vi "proc_get_exit_code.vi"(8 "error in":errorcluster, 10 "ignore error":bool=TRUE, 11 "process instance handle in":u32[](array[numeric])) -> (0 "error out":errorcluster, 1 "exited":bool, 2 "exit code":i32, 3 "process instance handle out":u32[](array[numeric]), 5 "running":bool)   [LabVIEW 2011]
doc: "Tries to read process instance exit code. Error is returned if process instance has not exited yet and STILL_ACTIVE (259) value is returned as an exit code.\nOptionally STILL_ACTIVE error can be filtered by 'ignore error' input (default)."
panel:
  in  "code mem":i32
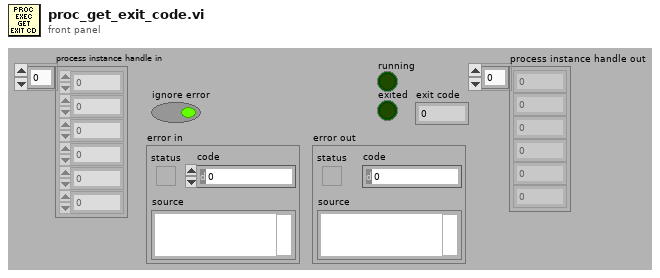
[diagram p1: front panel]
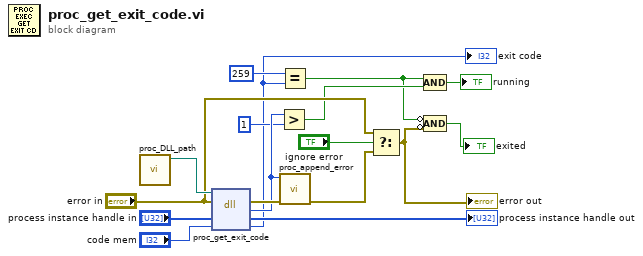
[diagram p0: block diagram]
diagram:
  n1 = call "proc_DLL_path.vi"() -> ("path out"=w17:path)  [unwired: 10 in, 1 out]
  n2 = dll-call lib="lv_proc.dll" fn="proc_get_exit_code"(path in=w17, error in="error in", "proc"="process instance handle in", "code"="code mem") -> (error out=w15:errorcluster, "error"=w11:i32, "proc"=→"process instance handle out":u32[], "code"=w2:i32)  [unwired: 1 in, 1 out]
  "exit code" <- w2
  n3 = Greater?(x=w11, y=1 ("x")) -> (0:w9:bool)
  n4 = Equal?(x=259, y=w2) -> (x = y?=w5:bool)
  n5 = call "proc_append_error.vi"("error in"=w15, "code in"=w11) -> ("error out"=w13:errorcluster)  [unwired: 8 in, 1 out]
  n6 = Select(t="error in", s="ignore error", f=w13) -> (s? t:f=w7:errorcluster)
  "error out" <- w7
  n7 = Compound Arithmetic op=AND(w5, w9) -> (→"running":bool)
  n8 = Compound Arithmetic op=AND(invert w5, invert w7) -> (→"exited":bool)
